vi "USB6343_Control_v1.3.vi"   [LabVIEW 2013]
uses:
  <vilib>/DAQmx/read.llb/DAQmx Read (Digital 1D Bool NChan 1Samp 1Line).vi
  <vilib>/DAQmx/read.llb/DAQmx Read (Analog 1D DBL NChan 1Samp).vi
  <vilib>/DAQmx/read.llb/DAQmx Read (Counter DBL 1Chan 1Samp).vi
  <vilib>/DAQmx/write.llb/DAQmx Write (Digital 1D Bool NChan 1Samp 1Line).vi
  <vilib>/DAQmx/write.llb/DAQmx Write (Analog 1D DBL NChan 1Samp).vi
  <vilib>/DAQmx/miscellaneous.llb/DAQmx Fill In Error Info.vi
types:
  T1 = cluster{"source":string, "channel":i32, "old value":dbl, "new value":dbl, "on/off":bool}
  T2 = cluster{"cmd":string, "channel":i32, "value":dbl, "on/off":bool, "return value":refnum<vi>}
  T3 = cluster{"AI Task":refnum<k21>, "AO Task":refnum<k21>, "DO Task":refnum<k21>, "DI Task":refnum<k21>}
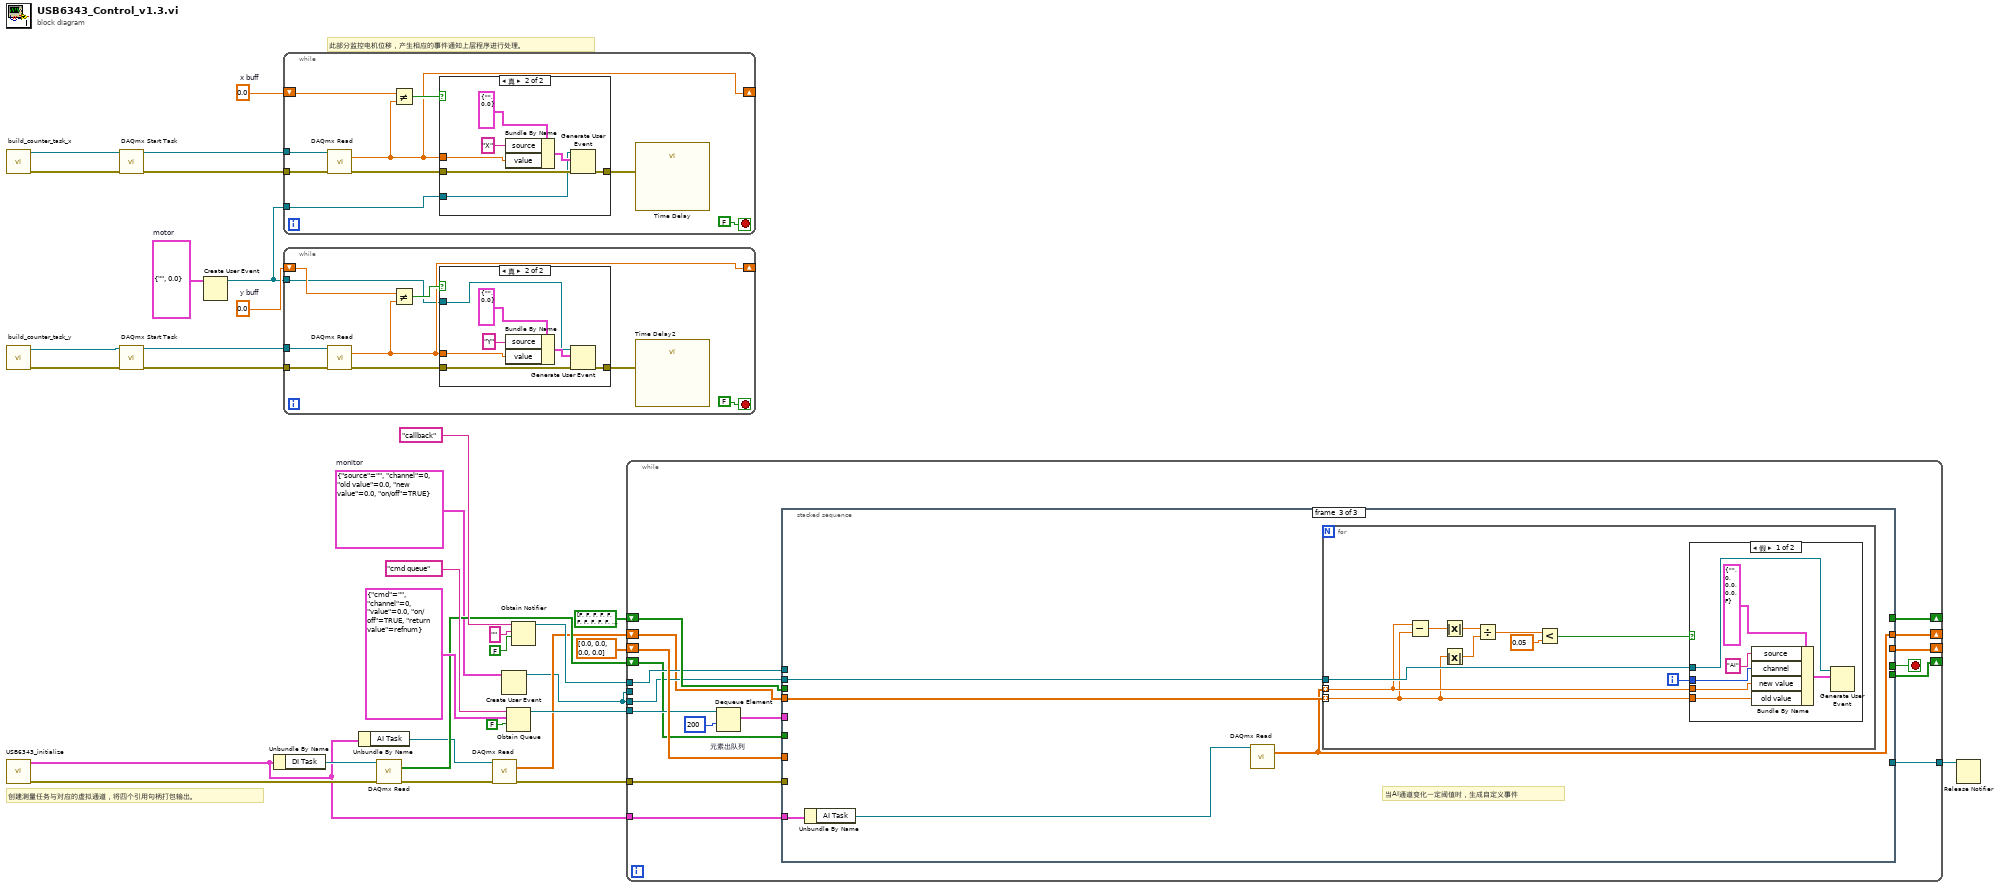
[diagram p0: block diagram]
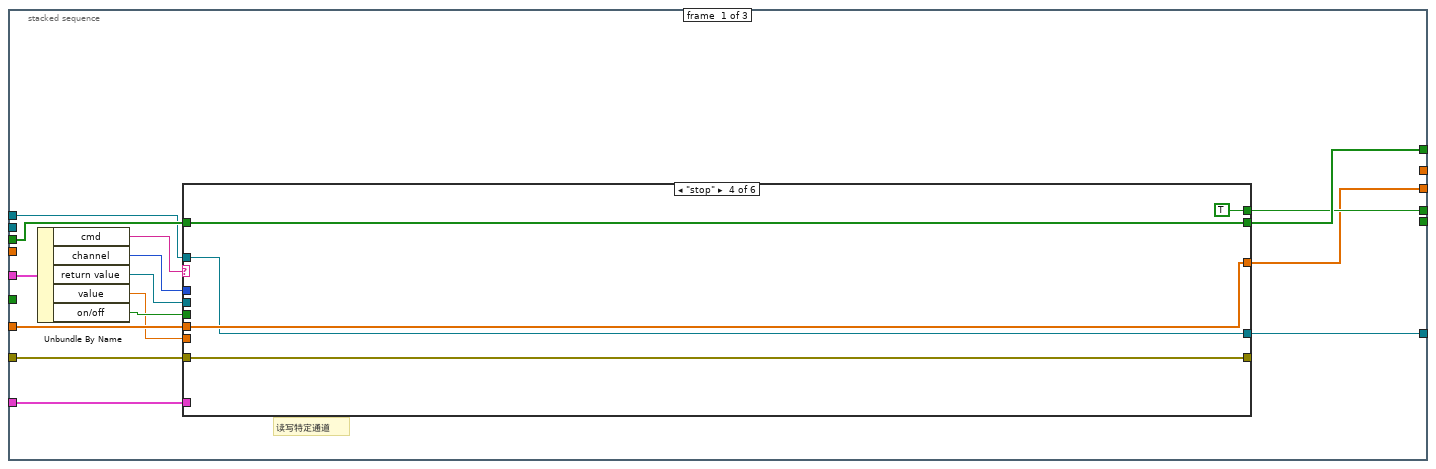
[diagram p4: hidden frame]
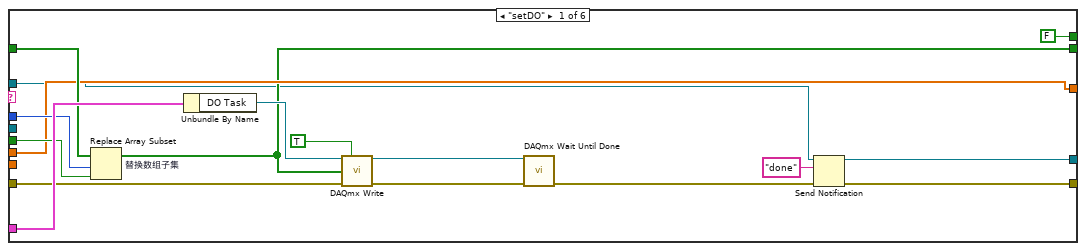
[diagram p5: hidden frame]
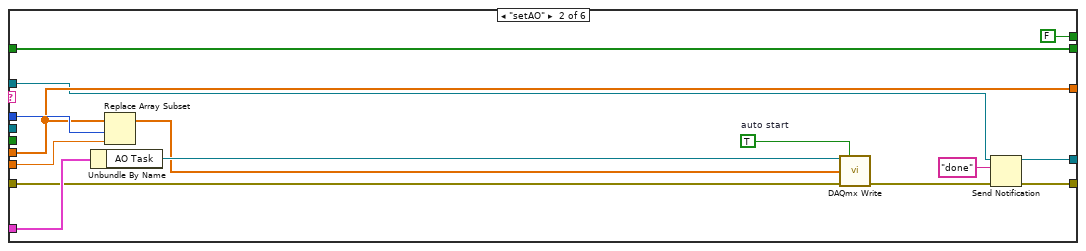
[diagram p6: hidden frame]
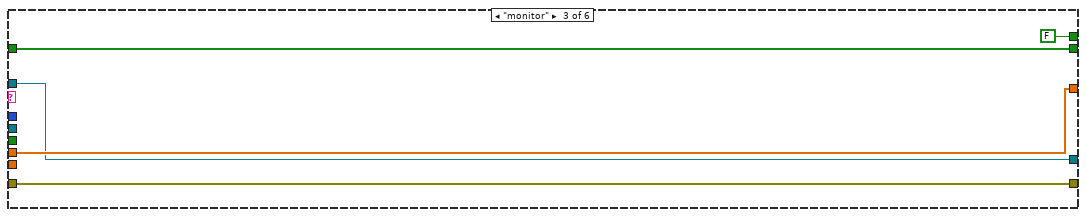
[diagram p7: hidden frame]
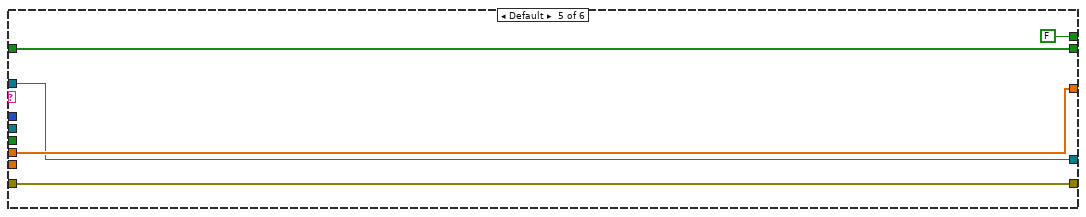
[diagram p8: hidden frame]
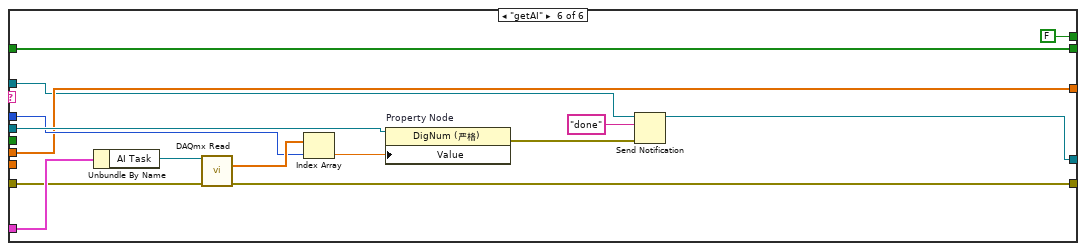
[diagram p9: hidden frame]
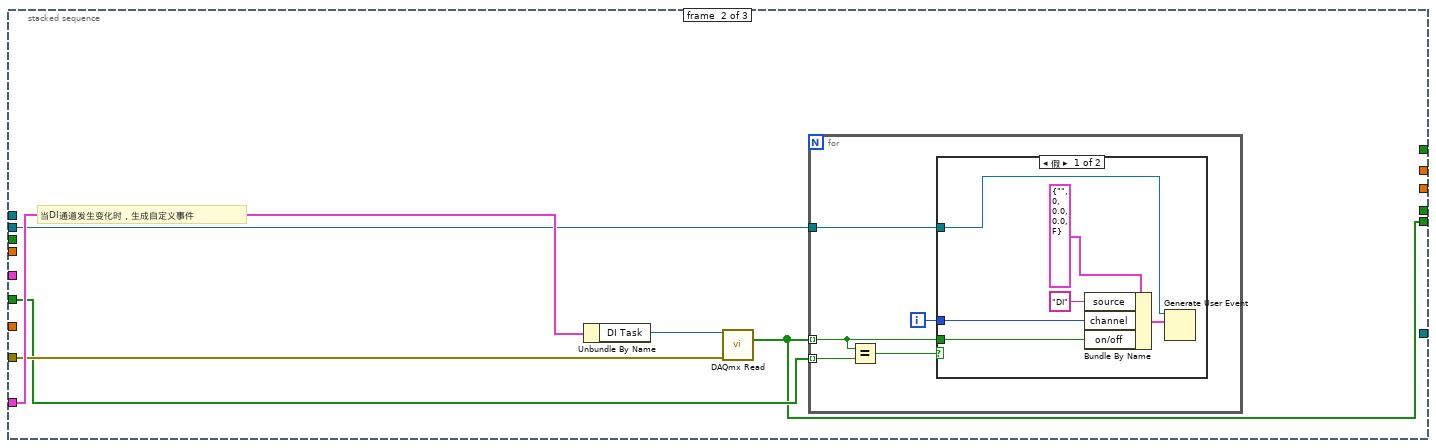
[diagram p10: hidden frame]
diagram:
  w2 = cluster{"source":string, "value":dbl} {"source"="", "value"=0.0}  # motor
  w4 = T1 {"source"="", "channel"=0, "old value"=0.0, "new value"=0.0, "on/off"=TRUE}  # monitor
  w26 = 0.0  # x buff
  w29 = 0.0  # y buff
  # "此部分监控电机位移，产生相应的事件通知上层程序进行处理。"
  # "创建测量任务与对应的虚拟通道，将四个引用句柄打包输出。"
  n1 = call "build_counter_task_x.vi"() -> ("error out"=w25:errorcluster, "task out"=w24:refnum<k21>)  [unwired: 10 in]
  n2 = call "build_counter_task_y.vi"() -> ("error out"=w22:errorcluster, "task out"=w23:refnum<k21>)  [unwired: 10 in]
  n3 = call "USB6343_initialize.vi"() -> ("error out"=w10:errorcluster, "tasks"=w7:T3)  [unwired: 10 in]
  n4 = call <vilib>:"DAQmx Start Task.vi"("task/channels in"=w24, "error in"=w25) -> ("task out"=w28:refnum<k21>, "error out"=w27:errorcluster)  [unwired: 12 in]
  n5 = call <vilib>:"DAQmx Start Task.vi"("task/channels in"=w23, "error in"=w22) -> ("task out"=w31:refnum<k21>, "error out"=w30:errorcluster)  [unwired: 12 in]
  n6 = Create User Event(user event datatype=w2) -> (user event=w1:refnum<user-event>)  [unwired: 1 in, 1 out]
  n7 = Unbundle By Name(w7) -> ("DI Task"=w12:refnum<k21>)
  n8 = while {
    tunnel: w28 -> [w40]
    tunnel: w27 -> [w42]
    shift-right: [w38] -> _
    shift-left: w26 -> [w41]
    tunnel: w1 -> [w34]
    stop <- FALSE stop-if-true
    n9 = call-poly <vilib>:"DAQmx Read.vi"("task/channels in"=w40, "error in"=w42) -> ("data"=w38:dbl, "error out"=w37:errorcluster)  [unwired: 11 in, 1 out]
    n10 = Not Equal?(x=w41, y=w38) -> (x != y?=w39:bool)
    n11 = case shown="真" w39 {
      tunnel: w38 -> [_ w48]
      tunnel: w37 -> [w43 w46]
      tunnel: [w43 w45] -> w35
      tunnel: w34 -> [_ w44]
      frame False {
      }
      frame True {
        n12 = Bundle By Name(cluster=cluster{"source":string, "value":dbl} {"source"="", "value"=0.0} ("事件数据"), "source"="X", "value"=w48) -> (w47:cluster{"source":string, "value":dbl})
        n13 = Generate User Event(user event=w44, event data cluster=w47, error in=w46) -> (error out=w45:errorcluster)  [unwired: 1 in, 1 out]
      }
    }
    n14 = call "Time Delay"("error in (no error)"=w35) -> ()  [unwired: 10 in, 1 out]
  }
  n15 = while {
    tunnel: w31 -> [w57]
    tunnel: w30 -> [w59]
    shift-right: [w55] -> _
    shift-left: w29 -> [w58]
    tunnel: w1 -> [w51]
    stop <- FALSE stop-if-true
    n16 = call-poly <vilib>:"DAQmx Read.vi"("task/channels in"=w57, "error in"=w59) -> ("data"=w55:dbl, "error out"=w54:errorcluster)  [unwired: 11 in, 1 out]
    n17 = Not Equal?(x=w58, y=w55) -> (x != y?=w56:bool)
    n18 = case shown="真" w56 {
      tunnel: w55 -> [_ w61]
      tunnel: w54 -> [w60 w63]
      tunnel: [w60 w62] -> w52
      tunnel: w51 -> [_ w64]
      frame False {
      }
      frame True {
        n19 = Bundle By Name(cluster=cluster{"source":string, "value":dbl} {"source"="", "value"=0.0} ("事件数据"), "source"="Y", "value"=w61) -> (w65:cluster{"source":string, "value":dbl})
        n20 = Generate User Event(user event=w64, event data cluster=w65, error in=w63) -> (error out=w62:errorcluster)  [unwired: 1 in, 1 out]
      }
    }
    n21 = call "Time Delay2"("error in (no error)"=w52) -> ()  [unwired: 10 in, 1 out]
  }
  n22 = Unbundle By Name(w7) -> ("AI Task"=w6:refnum<k21>)
  n23 = call-poly <vilib>:"DAQmx Read.vi"("task/channels in"=w12, "error in"=w10) -> ("data"=w11:bool[], "error out"=w9:errorcluster)  [unwired: 11 in, 1 out]
  n24 = call-poly <vilib>:"DAQmx Read.vi"("task/channels in"=w6, "error in"=w9) -> ("data"=w5:dbl[], "error out"=w8:errorcluster)  [unwired: 11 in, 1 out]
  n25 = Create User Event(user event datatype=w4) -> (user event=w3:refnum<user-event>)  [unwired: 1 in, 1 out]
  n26 = Obtain Queue(name (unnamed)="cmd queue" ("名称（未命名）"), element data type=T2 {"cmd"="", "channel"=0, "value"=0.0, "on/off"=TRUE, "return value"=refnum}, create if not found? (T)=FALSE ("如未找到是否创建？(T)")) -> (queue out=w19:refnum<queue>)  [unwired: 2 in, 2 out]
  n27 = Obtain Notifier(name (unnamed)="callback" ("名称（未命名）"), notification data type="", create if not found? (T)=FALSE ("如未找到是否创建？(T)")) -> (notifier out=w15:refnum<notifier>)  [unwired: 1 in, 2 out]
  n28 = while {
    tunnel: w7 -> [w78]
    tunnel: w8 -> [w84]
    shift-right: [w82] -> _
    shift-left: bool[] [FALSE, FALSE, FALSE, FALSE, FALSE, FALSE, FALSE, FALSE, FALSE, FALSE, FALSE, FALSE, FALSE, FALSE, FALSE, FALSE] -> [w83]
    shift-right: [w79] -> _
    shift-left: dbl[] [0.0, 0.0, 0.0, 0.0] ("data") -> [w80]
    tunnel: w19 -> [w77]
    tunnel: w15 -> [w74]
    tunnel: [w73] -> w14
    shift-right: [w71] -> _
    shift-left: w11 -> [w72]
    shift-right: [w68] -> _
    shift-left: w5 -> [w69]
    tunnel: w3 -> [w70]
    tunnel: w3 -> [_]
    stop <- w81 stop-if-true
    n29 = Dequeue Element "元素出队列"(queue=w77, timeout in ms (-1)=200 ("超时毫秒(-1)")) -> (element=w76:T2)  [unwired: 1 in, 3 out]
    n30 = stacked-sequence {
      tunnel: w84 -> [w99 w165 _]
      tunnel: w83 -> [w98 _ _]
      tunnel: [w97 _ _] -> w82
      tunnel: [w96 _ _] -> w81
      tunnel: w80 -> [w95 _ _]
      tunnel: [w94 _ _] -> w79
      tunnel: w78 -> [w85 w167 w183]
      tunnel: w76 -> [w93 _ _]
      tunnel: w74 -> [w87 _ _]
      tunnel: [w86 _ _] -> w73
      tunnel: w72 -> [_ w164 _]
      tunnel: [_ w163 _] -> w71
      tunnel: w70 -> [_ w162 w179]
      tunnel: w69 -> [_ _ w181]
      tunnel: [_ _ w180] -> w68
      frame #0 {
        # "读写特定通道"
        n31 = Unbundle By Name(w93) -> ("cmd"=w92:string, "channel"=w91:i32, "return value"=w90:refnum<vi>, "value"=w88:dbl, "on/off"=w89:bool)
        n32 = case shown="\"stop\"" w92 {
          tunnel: w91 -> [w114 w129 _ _ _ w156]
          tunnel: w85 -> [w116 w131 _ _ _ w161]
          tunnel: w99 -> [w108 w123 w133 w138 w143 w158]
          tunnel: w98 -> [w115 w127 w136 w141 w146 w154]
          tunnel: w89 -> [w113 _ _ _ _ _]
          tunnel: [w106 w127 w136 w141 w146 w154] -> w97
          tunnel: [FALSE FALSE FALSE TRUE FALSE FALSE] -> w96
          tunnel: w95 -> [w111 w128 w135 w139 w144 w153]
          tunnel: [w111 w128 w135 w139 w144 w153] -> w94
          tunnel: w90 -> [_ _ _ _ _ w159]
          tunnel: [w110 w121 w133 w138 w143 w151] -> _
          tunnel: w88 -> [_ w119 _ _ _ _]
          tunnel: w87 -> [w101 w118 w132 w137 w142 w148]
          tunnel: [w100 w117 w132 w137 w142 w147] -> w86
          frame "setDO" {
            n33 = Replace Array Subset "替换数组子集"(array=w115, new element=w113, index=w114) -> (w106:bool[])
            n34 = Unbundle By Name(w116) -> ("DO Task"=w107:refnum<k21>)
            n35 = call-poly <vilib>:"DAQmx Write.vi"("task/channels in"=w107, "auto start"=TRUE, "data"=w106, "error in"=w108) -> ("task out"=w102:refnum<k21>, "error out"=w104:errorcluster)  [unwired: 9 in, 1 out]
            n36 = call <vilib>:"DAQmx Wait Until Done.vi"("task/channels in"=w102, "error in"=w104) -> ("error out"=w103:errorcluster)  [unwired: 12 in, 1 out]
            n37 = Send Notification(notification="done" ("通知"), notifier=w101, error in (no error)=w103) -> (notifier out=w100:refnum<notifier>, error out=w110:errorcluster)
          }
          frame "setAO" {
            w125 = TRUE  # auto start
            n38 = Unbundle By Name(w131) -> ("AO Task"=w130:refnum<k21>)
            n39 = Replace Array Subset(array=w128, new element=w119, index=w129) -> (w126:dbl[])
            n40 = call-poly <vilib>:"DAQmx Write.vi"("task/channels in"=w130, "auto start"=w125, "data"=w126, "error in"=w123) -> ("error out"=w122:errorcluster)  [unwired: 9 in, 2 out]
            n41 = Send Notification(notification="done" ("通知"), notifier=w118, error in (no error)=w122) -> (notifier out=w117:refnum<notifier>, error out=w121:errorcluster)
          }
          frame "monitor" {
          }
          frame "stop" {
          }
          frame Default {
          }
          frame "getAI" {
            n42 = Unbundle By Name(w161) -> ("AI Task"=w160:refnum<k21>)
            n43 = call-poly <vilib>:"DAQmx Read.vi"("task/channels in"=w160, "error in"=w158) -> ("data"=w157:dbl[], "error out"=w151:errorcluster)  [unwired: 11 in, 1 out]
            n44 = Index Array(array=w157, index=w156) -> (element=w155:dbl)
            n45 = property on="Property Node" class="DigNum (严格)"(reference=w159, "Value"=w155) -> (error out=w149:errorcluster)  [unwired: 1 in, 1 out]
            n46 = Send Notification(notification="done" ("通知"), notifier=w148, error in (no error)=w149) -> (notifier out=w147:refnum<notifier>)  [unwired: 1 out]
          }
        }
      }
      frame #1 {
        # "当DI通道发生变化时，生成自定义事件"
        n47 = Unbundle By Name(w167) -> ("DI Task"=w166:refnum<k21>)
        n48 = call-poly <vilib>:"DAQmx Read.vi"("task/channels in"=w166, "error in"=w165) -> ("data"=w163:bool[])  [unwired: 11 in, 2 out]
        n49 = for {
          tunnel: w163 -> [w168] mode=indexing
          tunnel: w164 -> [w172] mode=indexing
          tunnel: w162 -> [w169]
          i -> [w170]
          n50 = Equal?(x=w168, y=w172) -> (x = y?=w171:bool)
          n51 = case shown="假" w171 {
            tunnel: w170 -> [w175 _]
            tunnel: w169 -> [w178 _]
            tunnel: w168 -> [w174 _]
            frame False {
              n52 = Bundle By Name(cluster=T1 {"source"="", "channel"=0, "old value"=0.0, "new value"=0.0, "on/off"=FALSE} ("事件数据"), "source"="DI", "channel"=w175, "on/off"=w174) -> (w173:T1)
              n53 = Generate User Event(user event=w178, event data cluster=w173) -> ()  [unwired: 2 in, 2 out]
            }
            frame True {
            }
          }
        }
      }
      frame #2 {
        # "当AI通道变化一定阈值时，生成自定义事件"
        n54 = Unbundle By Name(w183) -> ("AI Task"=w182:refnum<k21>)
        n55 = call-poly <vilib>:"DAQmx Read.vi"("task/channels in"=w182) -> ("data"=w180:dbl[])  [unwired: 12 in, 2 out]
        n56 = for {
          tunnel: w180 -> [w185] mode=indexing
          tunnel: w181 -> [w184] mode=indexing
          tunnel: w179 -> [w187]
          i -> [w186]
          n57 = Subtract(x=w185, y=w184) -> (x-y=w193:dbl)
          n58 = Absolute Value(x=w193) -> (abs(x)=w192:dbl)
          n59 = Absolute Value(x=w184) -> (abs(x)=w191:dbl)
          n60 = Divide(x=w192, y=w191) -> (x/y=w190:dbl)
          n61 = Less?(x=w190, y=0.05) -> (x < y?=w188:bool)
          n62 = case shown="假" w188 {
            tunnel: w187 -> [w200 _]
            tunnel: w186 -> [w197 _]
            tunnel: w185 -> [w196 _]
            tunnel: w184 -> [w195 _]
            frame False {
              n63 = Bundle By Name(cluster=T1 {"source"="", "channel"=0, "old value"=0.0, "new value"=0.0, "on/off"=FALSE} ("事件数据"), "source"="AI", "channel"=w197, "new value"=w196, "old value"=w195) -> (w194:T1)
              n64 = Generate User Event(user event=w200, event data cluster=w194) -> ()  [unwired: 2 in, 2 out]
            }
            frame True {
            }
          }
        }
      }
    }
  }
  n65 = Release Notifier(notifier=w14) -> ()  [unwired: 2 in, 3 out]
